vi "Full Name.vi"(10 "error in (no error)":errorcluster, 11 "Config Element in":refnum<class "Config Element.lvclass">) -> (2 "error out":errorcluster, 3 "Full Name":string)   [LabVIEW 2020, in "CDM-Config.lvlib" / "Config Element.lvclass"]
uses:
  Config Element.lvclass
  Config Element.lvclass/Config Element.ctl
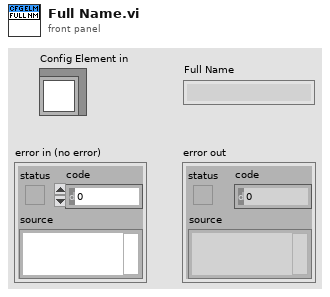
[diagram p1: front panel]
types:
  T1 = typedef "CDM-Config.lvlib/Config Element.lvclass/Ref Data.ctl" = cluster{"Config Element":T2, "Node Info":T4, "Owner":refnum<class>}
  T2 = typedef "CDM-Config.lvlib/Config Element.ctl" = cluster{"Full Name":string, "Name":string, "Value":string, "Meta Data":T3[]}
  T3 = typedef "CDM-Config.lvlib/Meta Data.ctl" = cluster{"Name":string, "Value":string}
  T4 = typedef "CDM-Config.lvlib/Node Info.ctl" = cluster{"Index":i32, "Parent":i32, "Children":i32[]}
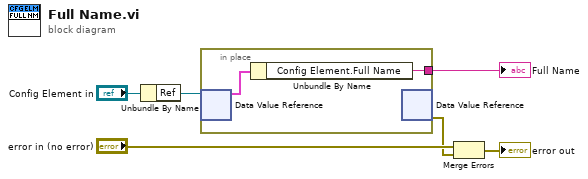
[diagram p0: block diagram]
diagram:
  n1 = Unbundle By Name("Config Element in") -> ("Ref"=w1:refnum<data-value>)
  n2 = in-place {
    in-place-border: [w7] -> w4
    n3 = in-place-dvr #1(w1) -> (w8:T1)  [unwired: 1 out]
    n4 = Unbundle By Name(w8) -> ("Config Element.Full Name"=w7:string)
    n5 = in-place-dvr #1() -> (w2:errorcluster)  [unwired: 1 in, 1 out]
  }
  "Full Name" <- w4
  n6 = Merge Errors("error in (no error)", w2) -> (→"error out":errorcluster)
